vi "rwfm_AcqReadTach.vi"(0 "FPGA VI Reference":refnum<k20>, 1 "Poll Time (ms)":u32=10, 5 "acq block size (s)":dbl=1.0 format="%#_13g", 9 "Samps Read per Chan":i32=-1, 11 "error in":errorcluster, 12 "Timeout (s)":dbl=5.0, 13 "OSClkStart":u32) -> (3 "OSClkStart":dbl, 4 "FPGA VI Reference Out":refnum<k20>, 8 "Tachometer Pulses":T1[](array[typedef]), 10 "Samples Remaining":u32, 14 "Read Time (ms)":u32, 15 "error out":errorcluster)   [LabVIEW 2017, in "cRIOWfmLib.lvlib"]
doc: "Reads waveform data from the DMA FIFO."
uses:
  <vilib>/addons/InsightCM/Devices/Shared/Cms/cRIOWfmAcq/cRIOWfmLib.lvlib
  <vilib>/addons/InsightCM/Utilities/Analysis/Shared/controls/PulsePositions.ctl
  <vilib>/addons/InsightCM/Utilities/Misc/rolloverState.ctl
  <vilib>/Utility/error.llb/Error Cluster From Error Code.vi
  <vilib>/rvi/errors/niLvFpgaAdjustHostInterfaceError.vi
  <vilib>/rvi/interface/nirviMethod/nirviMethod.xnode
  <vilib>/FPGAPlugInAG/Dynamic/niLvFpga_ReadFifo_Dynamic.vi
  <vilib>/rvi/errors/niLvFpgaMergeErrorWithErrorCode.vi
  <vilib>/addons/InsightCM/Utilities/Analysis/Shared/AnalysisHelper.lvlib
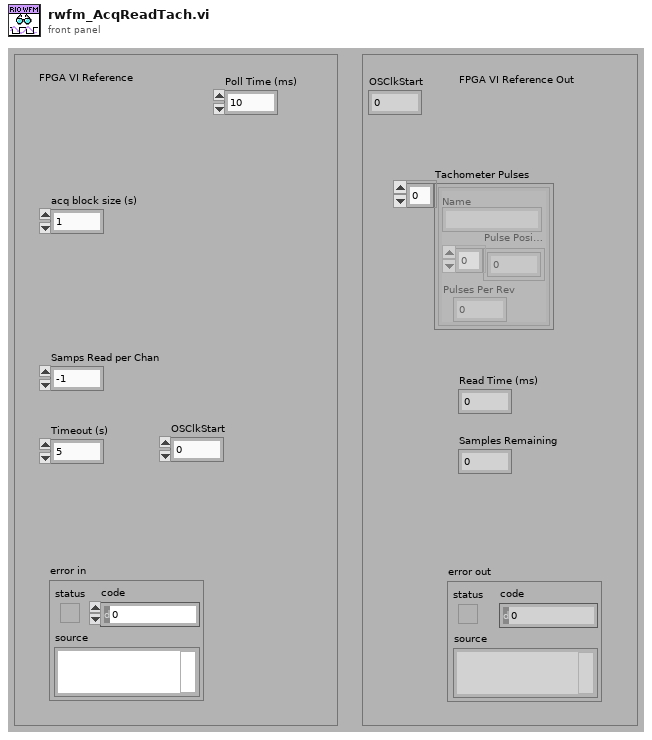
[diagram p1: front panel]
types:
  T1 = typedef "AnalysisHelper.lvlib/PulsePositions.ctl" = cluster{"Name":string, "Pulse Position Data":dbl[], "Pulses Per Rev":i32}
  T2 = typedef "rolloverState.ctl" = cluster{"prev value":u32, "total add":dbl}
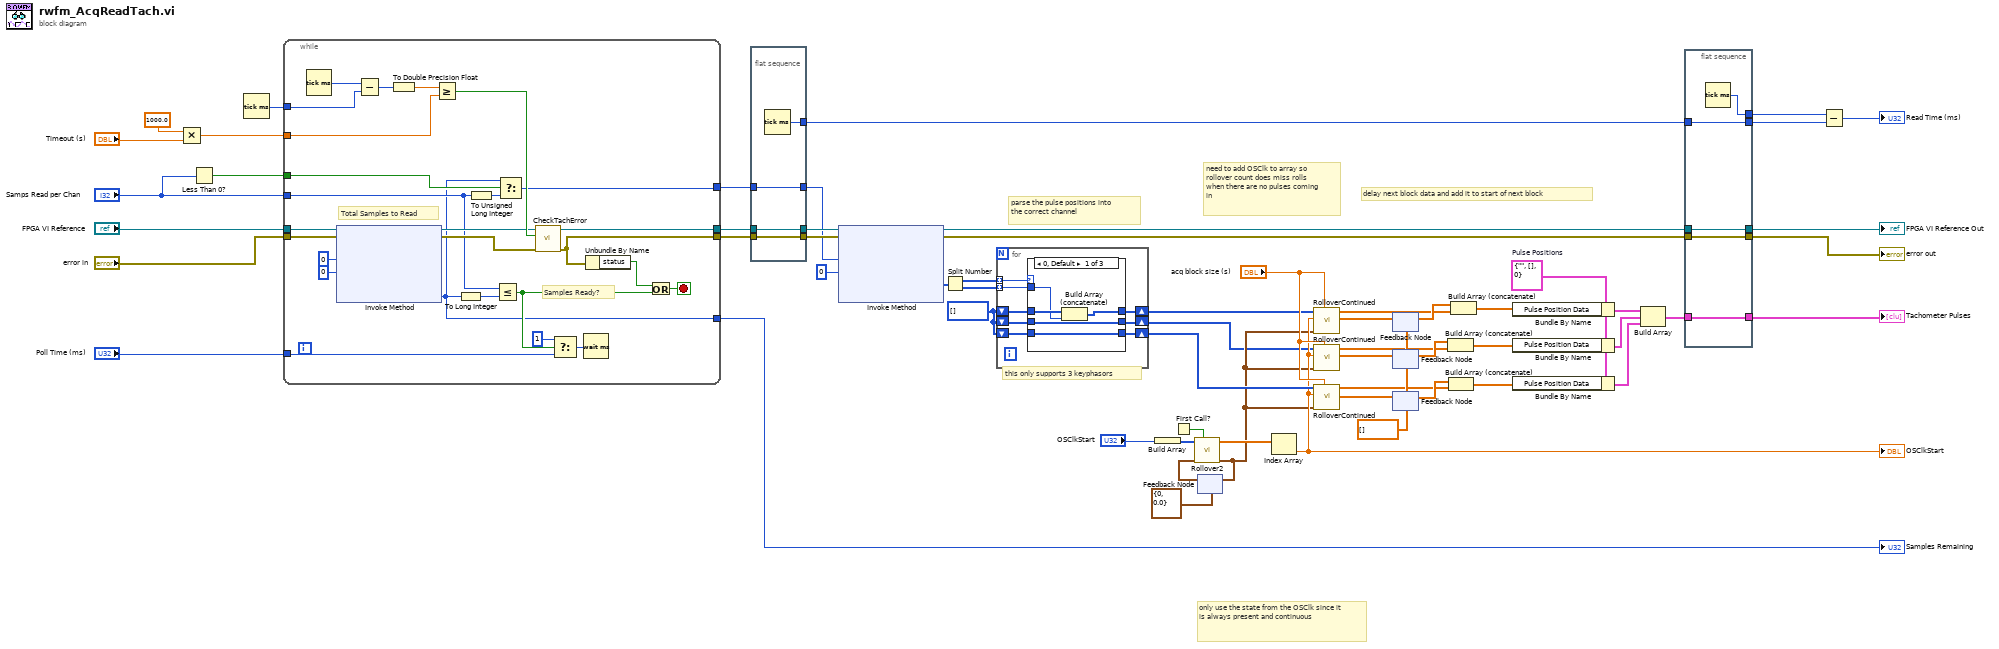
[diagram p0: block diagram]
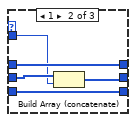
[diagram p2: hidden frame]
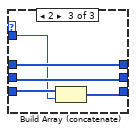
[diagram p3: hidden frame]
diagram:
  w4 = T1 {"Name"="", "Pulse Position Data"=[], "Pulses Per Rev"=0}  # Pulse Positions
  w15 = dbl[] [] ("next block")
  w33 = u32[] [] ("Data")
  # "delay next block data and add it to start of next block"
  # "only use the state from the OSClk since it is always present and continuous"
  # "need to add OSClk to array so rollover count does miss rolls when there are no pulses coming in"
  # "parse the pulse positions into the correct channel"
  # "this only supports 3 keyphasors"
  n1 = Multiply(x=1000.0 ("y"), y="Timeout (s)") -> (x*y=w41:dbl)
  n2 = Less Than 0?(x="Samps Read per Chan") -> (x < 0?=w38:bool)
  n3 = Tick Count (ms)() -> (millisecond timer value=w40:u32)
  n4 = while {
    tunnel: [w79] -> w44
    tunnel: [w65] -> w45
    tunnel: "FPGA VI Reference" -> [w73]
    tunnel: "error in" -> [w72]
    tunnel: w40 -> [w82]
    tunnel: w41 -> [w81]
    tunnel: "Poll Time (ms)" -> [w75]
    tunnel: [w69] -> w46
    tunnel: "Samps Read per Chan" -> [w62]
    tunnel: w38 -> [w68]
    tunnel: [w61] -> w3
    stop <- w85 stop-if-true
    # "Total Samples to Read"
    # "Samples Ready?"
    n5 = Tick Count (ms)() -> (millisecond timer value=w80:u32)
    n6 = xnode "Invoke Method"("FPGA VI Reference In"=w73, "error in"=w72, "Number of Elements"=u32 0, "Timeout (ms)"=0) -> ("FPGA VI Reference Out"=w67:refnum<k20>, "error out"=w66:errorcluster, "Elements Remaining"=w61:u32)  [unwired: 1 out]
    n7 = Subtract(x=w80, y=w82) -> (x-y=w84:u32)
    n8 = To Double Precision Float(number=w84) -> (double precision float=w83:dbl)
    n9 = Greater Or Equal?(x=w83, y=w81) -> (x >= y?=w78:bool)
    n10 = To Long Integer(number=w61) -> (32bit integer=w64:i32)
    n11 = To Unsigned Long Integer(number=w62) -> (unsigned 32bit integer=w63:u32)
    n12 = Less Or Equal?(x=w62, y=w64) -> (x <= y?=w76:bool)
    n13 = Select(t=w61, s=w68, f=w63) -> (s? t:f=w69:u32)
    n14 = call <vilib>:"CheckTachError.vi"("error in (no error)"=w66, "timeout"=w78, "fpga vi reference in"=w67) -> ("error out"=w79:errorcluster, "fpga vi reference out"=w65:refnum<k20>)  [unwired: 7 in]
    n15 = Select(t=u32 1, s=w76, f=w75) -> (s? t:f=w77:u32)
    n16 = Wait (ms)(milliseconds to wait=w77) -> ()  [unwired: 1 out]
    n17 = Unbundle By Name(w79) -> ("status"=w86:bool)
    n18 = Or(x=w86, y=w76) -> (x .or. y?=w85:bool)
  }
  "Samples Remaining" <- w3
  n19 = flat-sequence {
    tunnel: [w90] -> w50
    tunnel: w44 -> [w90]
    tunnel: [w89] -> w49
    tunnel: w45 -> [w89]
    tunnel: [w88] -> w48
    tunnel: w46 -> [w88]
    tunnel: [w87] -> w47
    frame #0 {
      n20 = Tick Count (ms)() -> (millisecond timer value=w87:u32)
    }
  }
  n21 = xnode "Invoke Method"("FPGA VI Reference In"=w49, "error in"=w50, "Number of Elements"=w48, "Timeout (ms)"=0) -> ("FPGA VI Reference Out"=w57:refnum<k20>, "error out"=w55:errorcluster, "Data"=w36:u64[])  [unwired: 1 out]
  n22 = Split Number(x=w36) -> (hi(x)=w35:u32[], lo(x)=w34:u32[])
  n23 = for {
    tunnel: w35 -> [w98] mode=indexing
    tunnel: w34 -> [w96] mode=indexing
    shift-right: [w93] -> w6
    shift-left: w33 -> [w97]
    shift-right: [w92] -> w2
    shift-left: w33 -> [w95]
    shift-right: [w91] -> w25
    shift-left: w33 -> [w94]
    n24 = case shown="0, Default" w98 {
      tunnel: w97 -> [w103 w108 w113]
      tunnel: w96 -> [w102 w106 w109]
      tunnel: w95 -> [w100 w107 w112]
      tunnel: w94 -> [w99 w104 w111]
      tunnel: [w101 w108 w113] -> w93
      tunnel: [w100 w105 w112] -> w92
      tunnel: [w99 w104 w110] -> w91
      frame 0, Default {
        n25 = Build Array (concatenate)(w103, w102) -> (w101:u32[])
      }
      frame 1 {
        n26 = Build Array (concatenate)(w107, w106) -> (w105:u32[])
      }
      frame 2 {
        n27 = Build Array (concatenate)(w111, w109) -> (w110:u32[])
      }
    }
  }
  n28 = Build Array("OSClkStart") -> (w23:u32[])
  n29 = First Call?() -> (First Call?: T/F=w26:bool)
  n30 = feedback #1(T2 {"prev value"=0, "total add"=0.0} ("rollover state")) -> (w22:T2)
  n31 = call <vilib>:"Rollover2.vi"("reset"=w26, "rollover state"=w22, "counter"=w23) -> ("rollover state"=w5:T2, "counter"=w27:dbl[])  [unwired: 7 in]
  n32 = feedback-in #1(w5) -> ()
  n33 = Index Array(array=w27) -> (element=w7:dbl)  [unwired: 1 in]
  "OSClkStart" <- w7
  n34 = call <vilib>:"RolloverContinued.vi"("acq block size (s)"="acq block size (s)", "rollover state"=w5, "OSClkStart"=w7, "counter"=w6) -> ("next block"=w8:dbl[], "this block"=w20:dbl[])  [unwired: 4 in, 2 out]
  n35 = call <vilib>:"RolloverContinued.vi"("acq block size (s)"="acq block size (s)", "rollover state"=w5, "OSClkStart"=w7, "counter"=w2) -> ("next block"=w17:dbl[], "this block"=w12:dbl[])  [unwired: 4 in, 2 out]
  n36 = call <vilib>:"RolloverContinued.vi"("acq block size (s)"="acq block size (s)", "rollover state"=w5, "OSClkStart"=w7, "counter"=w25) -> ("next block"=w16:dbl[], "this block"=w10:dbl[])  [unwired: 4 in, 2 out]
  n37 = feedback-in #2(w8) -> ()
  n38 = feedback #2(w15) -> (w21:dbl[])
  n39 = feedback #3(w15) -> (w13:dbl[])
  n40 = feedback-in #3(w17) -> ()
  n41 = feedback #4(w15) -> (w11:dbl[])
  n42 = feedback-in #4(w16) -> ()
  n43 = Build Array (concatenate)(w13, w12) -> (w14:dbl[])
  n44 = Build Array (concatenate)(w11, w10) -> (w9:dbl[])
  n45 = Build Array (concatenate)(w21, w20) -> (w19:dbl[])
  n46 = Bundle By Name(cluster=w4, "Pulse Position Data"=w19) -> (w32:T1)
  n47 = Bundle By Name(cluster=w4, "Pulse Position Data"=w14) -> (w31:T1)
  n48 = Bundle By Name(cluster=w4, "Pulse Position Data"=w9) -> (w30:T1)
  n49 = Build Array(w32, w31, w30) -> (w29:T1[])
  n50 = flat-sequence {
    tunnel: [w118] -> w56
    tunnel: w57 -> [w118]
    tunnel: [w117] -> w54
    tunnel: w55 -> [w117]
    tunnel: [w116] -> w53
    tunnel: [w115] -> w51
    tunnel: w47 -> [w115]
    tunnel: w29 -> [w114]
    tunnel: [w114] -> w1
    frame #0 {
      n51 = Tick Count (ms)() -> (millisecond timer value=w116:u32)
    }
  }
  n52 = Subtract(x=w53, y=w51) -> (x-y=→"Read Time (ms)":u32)
  "error out" <- w54
  "FPGA VI Reference Out" <- w56
  "Tachometer Pulses" <- w1
